vi "界面判断显示.vi"(7 "parameter IN":T1, 8 "FailNumber":string, 9 "PassNumber":string, 10 "Status":string, 11 "Image In":T2(plugin-control)) -> (0 "pass":string, 1 "fail":string, 3 "Image Out":T2(plugin-control), 4 "结果":bool, 5 "parameter oUT":T1)   [LabVIEW 2015]
panel:
  in  "3 Pause Message":string
  in  "2 Pause Message":string
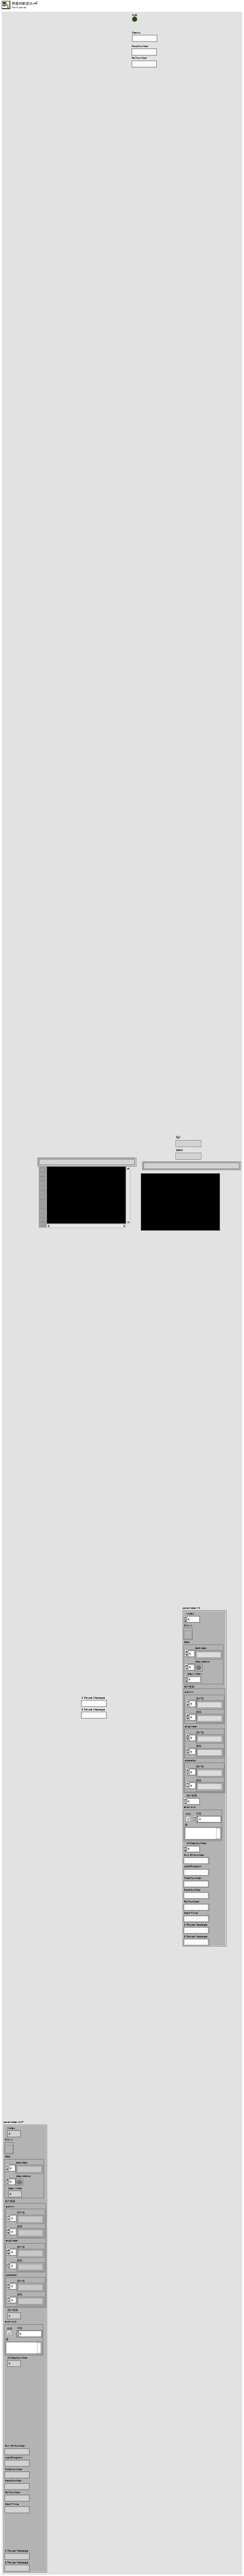
[diagram p1: front panel]
types:
  T1 = cluster{"index":i32, "this vi":refnum<vi>, "step":cluster{"test step":string[], "step status":bool[], "step index":i32}, "用户登录":cluster{"admin":cluster{"用户名":string[], "密码":string[]}, "engineer":cluster{"用户名":string[], "密码":string[]}, "operator":cluster{"用户名":string[], "密码":string[]}}, "用户权限":i32, "error out":errorcluster, "AllStepNumber":i32, "Run ErrNumber":string, "LoadProgram":string, "TotalNumber":string, "PassNumber":string, "FailNumber":string, "Start Time":string, "2 Pause Message":string, "3 Pause Message":string}
  T2 = typedef "IMAQ Image.ctl" = refnum<image>
  T3 = cluster{"Cent X":dbl, "Cent Y":dbl, "Big1 R":dbl, "Small1 R":dbl, "Big2 R":dbl, "Small2 R":dbl, "pass":dbl, "fail":dbl}
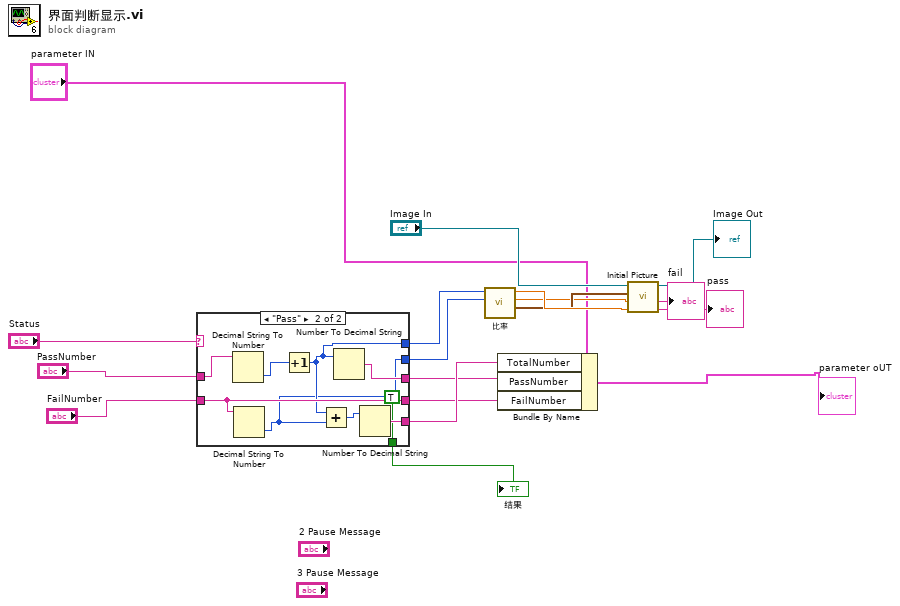
[diagram p0: block diagram]
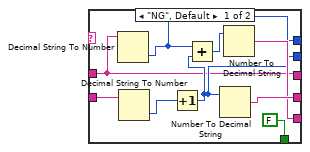
[diagram p2: hidden frame]
diagram:
  n1 = case shown="\"Pass\"" "Status" {
    tunnel: "PassNumber" -> [w19 w36]
    tunnel: "FailNumber" -> [w26 w33]
    tunnel: [w21 w32] -> w15
    tunnel: [w19 w34] -> w11
    tunnel: [w25 w33] -> w12
    tunnel: [w23 w30] -> w13
    tunnel: [w22 w29] -> w14
    tunnel: [FALSE TRUE] -> w3
    frame "NG", Default {
      n2 = Decimal String To Number(string=w19) -> (number=w21:i32)  [unwired: 2 in, 1 out]
      n3 = Decimal String To Number(string=w26) -> (number=w27:i32)  [unwired: 2 in, 1 out]
      n4 = Increment(x=w27) -> (x+1=w22:i32)
      n5 = Add(x=w21, y=w22) -> (x+y=w24:i32)
      n6 = Number To Decimal String(number=w22) -> (decimal integer string=w25:string)  [unwired: 1 in]
      n7 = Number To Decimal String(number=w24) -> (decimal integer string=w23:string)  [unwired: 1 in]
    }
    frame "Pass" {
      n8 = Decimal String To Number(string=w36) -> (number=w35:i32)  [unwired: 2 in, 1 out]
      n9 = Decimal String To Number(string=w33) -> (number=w29:i32)  [unwired: 2 in, 1 out]
      n10 = Increment(x=w35) -> (x+1=w32:i32)
      n11 = Add(x=w32, y=w29) -> (x+y=w31:i32)
      n12 = Number To Decimal String(number=w32) -> (decimal integer string=w34:string)  [unwired: 1 in]
      n13 = Number To Decimal String(number=w31) -> (decimal integer string=w30:string)  [unwired: 1 in]
    }
  }
  "结果" <- w3
  n14 = call "比率.vi"("Fail 个数"=w14, "Pass 个数"=w15) -> ("result"=w8:T3, "fail 率"=w7:dbl, "pass率"=w9:dbl)  [unwired: 7 in]
  n15 = Bundle By Name(cluster="parameter IN", "TotalNumber"=w13, "PassNumber"=w11, "FailNumber"=w12) -> (→"parameter oUT":T1)
  n16 = call "Initial Picture.vi"("Pass"=w9, "fail"=w7, "中心位置"=w8, "Image In"="Image In") -> ("pass"=→"pass":string, "fail"=→"fail":string, "Image Out"=→"Image Out":T2)  [unwired: 4 in, 1 out]
